vi "Additional Installer to SBOM Component.vi"(8 "error in (no error)":errorcluster, 11 "Additional Installer":T1={"flavorID"="DefaultFull", "productID"="{1A4448CF-1F95-420D-ABAD-2AB572A8A341}", "productName"="NI LabVIEW Runtime 2017 SP1 f3", "upgradeCode"="{620DBAE1-B159-4204-8186-0813C8A6434C}", "SoftDeps"=[{"productName"="NI LabVIEW Runtime 2017 SP1 Non-English Support.", "upgradeCode"="{182AE811-85B6-4238-B67E-F19497CC186B}", "exclude?"=FALSE}, {"productName"="NI ActiveX Container", "upgradeCode"="{1038A887-23E1-4289-B0BD-0C4B83C6BA21}", "exclude?"=FALSE}, {"productName"="Math Kernel Libraries", "upgradeCode"="{699C1AC5-2CF2-4745-9674-B19536EBA8A3}", "exclude?"=FALSE}, {"productName"="NI Logos 18.0", "upgradeCode"="{5E4A4CE3-4D06-11D4-8B22-006008C16337}", "exclude?"=FALSE}, {"productName"="NI TDM Streaming 18.0", "upgradeCode"="{4CD11BE6-6BB7-4082-8A27-C13771BC309B}", "exclude?"=FALSE}, {"productName"="NI LabVIEW Web Server 2017", "upgradeCode"="{0960380B-EA86-4E0C-8B57-14CD8CCF2C15}", "exclude?"=FALSE}, {"productName"="NI LabVIEW Real-Time NBFifo 2017", "upgradeCode"="{4F261250-2C38-488D-A9EC-9D1EFCC24D4B}", "exclude?"=FALSE}, {"productName"="NI VC2008MSMs", "upgradeCode"="{FDA3F8BB-BAA9-45D7-8DC7-22E1F5C76315}", "exclude?"=FALSE}, {"productName"="NI VC2010MSMs", "upgradeCode"="{EFBA6F9E-F934-4BD7-AC51-60CCA480489C}", "exclude?"=FALSE}, {"productName"="NI VC2015 Runtime", "upgradeCode"="{D42E7BAE-6589-4570-B6A3-3E28889392E7}", "exclude?"=FALSE}, {"productName"="NI mDNS Responder 17.0", "upgradeCode"="{9607874B-4BB3-42CB-B450-A2F5EF60BA3B}", "exclude?"=FALSE}, {"productName"="NI Deployment Framework 2018", "upgradeCode"="{838942E4-B73C-492E-81A3-AA1E291FD0DC}", "exclude?"=FALSE}, {"productName"="NI Error Reporting 2018", "upgradeCode"="{42E818C6-2B08-4DE7-BD91-B0FD704C119A}", "exclude?"=FALSE}]}) -> (0 "error out":errorcluster, 3 "LabVIEW installer component out":refnum<class "CycloneDX Component.lvclass">)   [LabVIEW 2017, in "LabVIEW Installer Support.lvlib"]
doc: "Converts LabVIEW installer build specification 'additional installers' to a list of SBOM components"
uses:
  LabVIEW Installer Support.lvlib
  Additional Installer.ctl
  Installer Soft Dep.ctl
  CycloneDX/CycloneDX Component/CycloneDX Component.lvclass
  C:/LabVIEW Working Directory/labview-cyclonedx-sbom/Source/CycloneDX/CycloneDX JSON/CycloneDX JSON.lvclass
  CycloneDX/CycloneDX JSON/CycloneDX Types.ctl
  CycloneDX/CycloneDX JSON/CycloneDX JSON.lvclass
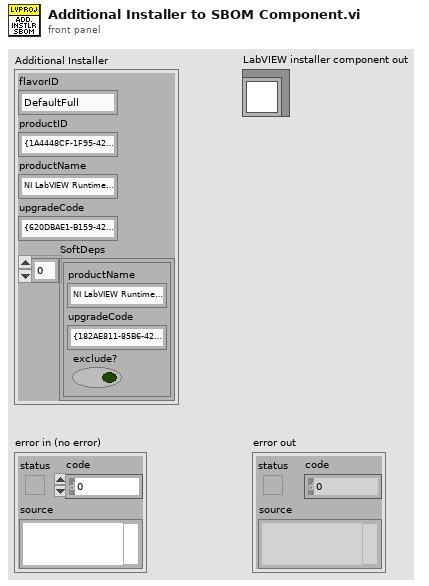
[diagram p1: front panel]
types:
  T1 = typedef "LabVIEW Installer Support.lvlib/Additional Installer.ctl" = cluster{"flavorID":string, "productID":string, "productName":string, "upgradeCode":string, "SoftDeps":T2[]}
  T2 = typedef "LabVIEW Installer Support.lvlib/Installer Soft Dep.ctl" = cluster{"productName":string, "upgradeCode":string, "exclude?":bool}
  T3 = typedef "LabVIEW CycloneDX SBOM.lvlib/CycloneDX JSON.lvclass/CycloneDX Types.ctl" = enum16{"application", "framework", "library", "container", "platform", "operating-system", "device", "device-driver", "firmware", "file", "machine-learning-model", "data"}
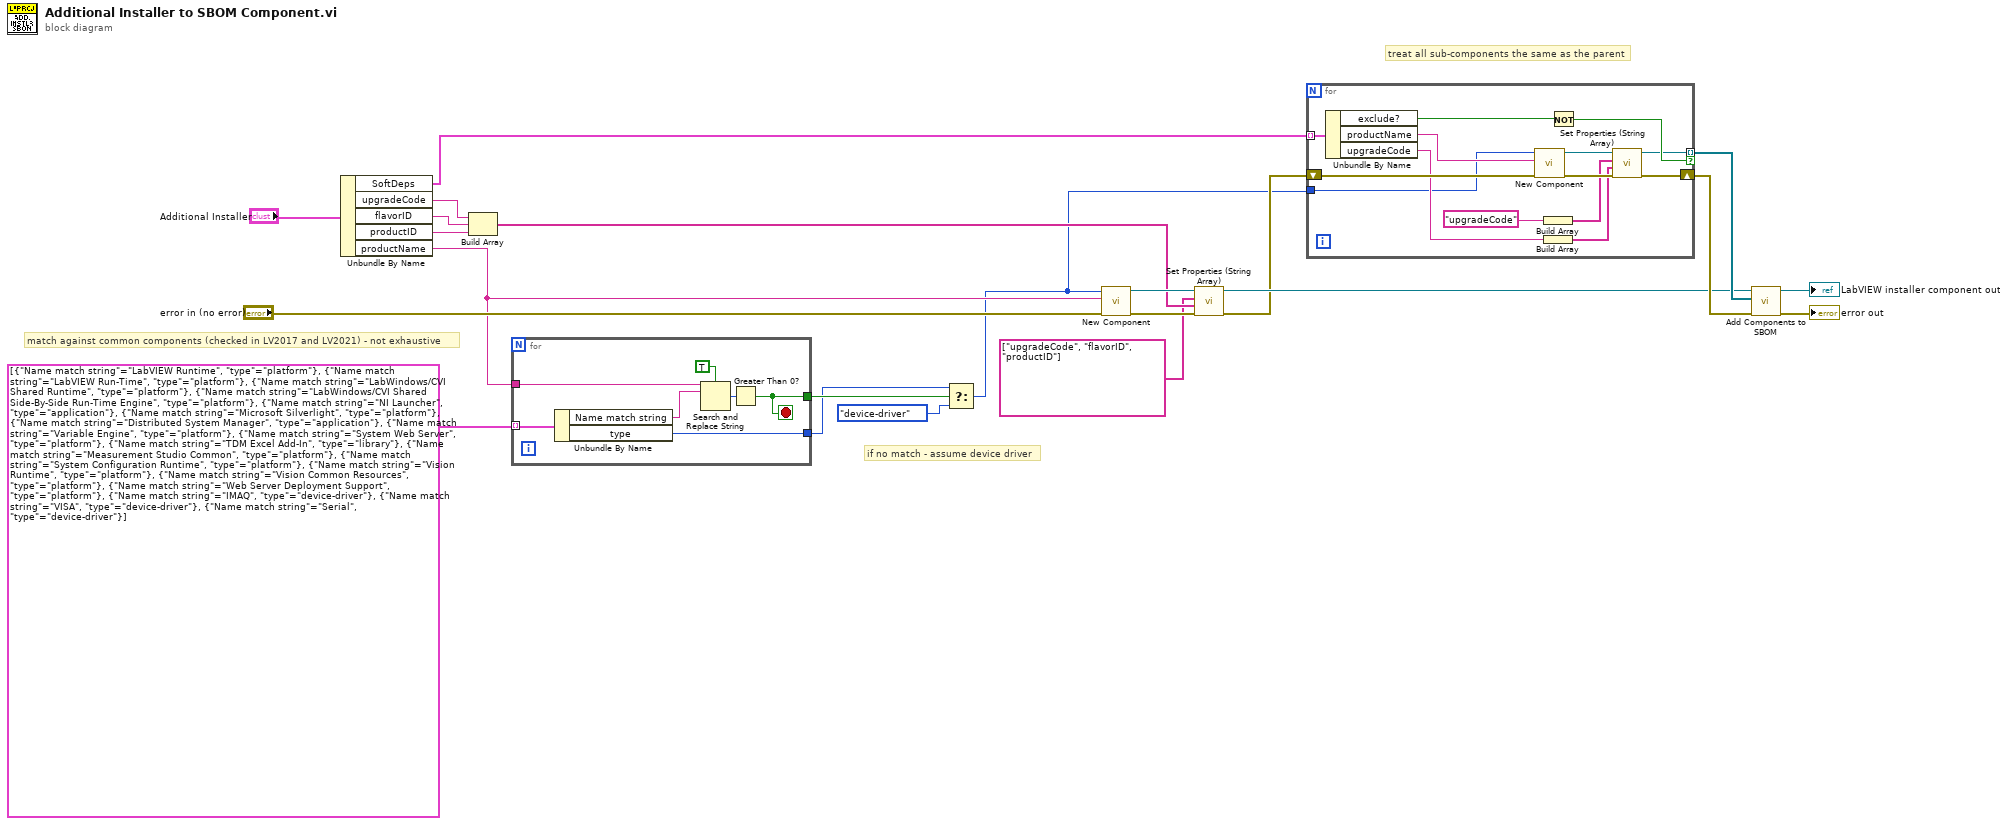
[diagram p0: block diagram]
diagram:
  # "match against common components (checked in LV2017 and LV2021) - not exhaustive"
  # "if no match - assume device driver"
  # "treat all sub-components the same as the parent"
  n1 = Unbundle By Name("Additional Installer") -> ("SoftDeps"=w16:T2[], "upgradeCode"=w11:string, "flavorID"=w10:string, "productID"=w9:string, "productName"=w5:string)
  n2 = Build Array(w11, w10, w9) -> (w8:string[])
  n3 = for {
    tunnel: cluster{"Name match string":string, "type":T3}[] [{"Name match string"="LabVIEW Runtime", "type"=enum."platform"}, {"Name match string"="LabVIEW Run-Time", "type"=enum."platform"}, {"Name match string"="LabWindows/CVI Shared Runtime", "type"=enum."platform"}, {"Name match string"="LabWindows/CVI Shared Side-By-Side Run-Time Engine", "type"=enum."platform"}, {"Name match string"="NI Launcher", "type"=enum."application"}, {"Name match string"="Microsoft Silverlight", "type"=enum."platform"}, {"Name match string"="Distributed System Manager", "type"=enum."application"}, {"Name match string"="Variable Engine", "type"=enum."platform"}, {"Name match string"="System Web Server", "type"=enum."platform"}, {"Name match string"="TDM Excel Add-In", "type"=enum."library"}, {"Name match string"="Measurement Studio Common", "type"=enum."platform"}, {"Name match string"="System Configuration Runtime", "type"=enum."platform"}, {"Name match string"="Vision Runtime", "type"=enum."platform"}, {"Name match string"="Vision Common Resources", "type"=enum."platform"}, {"Name match string"="Web Server Deployment Support", "type"=enum."platform"}, {"Name match string"="IMAQ", "type"=enum."device-driver"}, {"Name match string"="VISA", "type"=enum."device-driver"}, {"Name match string"="Serial", "type"=enum."device-driver"}] -> [w29] mode=indexing
    tunnel: w5 -> [w26]
    tunnel: [w24] -> w4
    tunnel: [w23] -> w3
    stop <- w24 stop-if-true
    n4 = Unbundle By Name(w29) -> ("Name match string"=w27:string, "type"=w23:T3)
    n5 = Search and Replace String(case sensitive?=TRUE ("ignore case? (F)"), input string=w26, search string=w27) -> (number of replacements=w25:i32)  [unwired: 5 in, 3 out]
    n6 = Greater Than 0?(x=w25) -> (x > 0?=w24:bool)
  }
  n7 = Select(t=w3, s=w4, f=CycloneDX_Types."device-driver") -> (s? t:f=w2:T3)
  n8 = call "New Component.vi"("error in (no error)"="error in (no error)", "name"=w5, "type"=w2) -> ("error out"=w14:errorcluster, "CycloneDX Component out"=w15:refnum<class "CycloneDX Component.lvclass">)  [unwired: 7 in]
  n9 = call "Set Properties (String Array).vi"("error in (no error)"=w14, "values (string)"=w8, "names"=string[] ["upgradeCode", "flavorID", "productID"], "CycloneDX JSON in"=w15) -> ("error out"=w12:errorcluster, "CycloneDX JSON out"=w13:refnum<class "CycloneDX Component.lvclass">)  [unwired: 6 in]
  n10 = for {
    tunnel: [w35] -> w18 mode=indexing if=w40
    shift-right: [w36] -> w17
    shift-left: w12 -> [w43]
    tunnel: w16 -> [w42] mode=indexing
    tunnel: w2 -> [w30]
    n11 = Unbundle By Name(w42) -> ("exclude?"=w41:bool, "productName"=w39:string, "upgradeCode"=w34:string)
    n12 = call "New Component.vi"("error in (no error)"=w43, "name"=w39, "type"=w30) -> ("error out"=w37:errorcluster, "CycloneDX Component out"=w38:refnum<class "CycloneDX Component.lvclass">)  [unwired: 7 in]
    n13 = Build Array("upgradeCode") -> (w31:string[])
    n14 = Build Array(w34) -> (w33:string[])
    n15 = Not(x=w41) -> (.not. x?=w40:bool)
    n16 = call "Set Properties (String Array).vi"("error in (no error)"=w37, "values (string)"=w33, "names"=w31, "CycloneDX JSON in"=w38) -> ("error out"=w36:errorcluster, "CycloneDX JSON out"=w35:refnum<class "CycloneDX Component.lvclass">)  [unwired: 6 in]
  }
  n17 = call "Add Components to SBOM.vi"("error in (no error)"=w17, "Component(s) to add"=w18, "CycloneDX SBOM in"=w13) -> ("error out"=→"error out":errorcluster, "CycloneDX SBOM out"=→"LabVIEW installer component out":refnum<class "CycloneDX Component.lvclass">)  [unwired: 7 in]
